vi "InsertNumArrIntoHashTbl.vi"(2 "Hash Table In":refnum<class "HashTable.lvclass">, 3 "Numeric Array In":i32[](array[numeric])) -> (0 "Hash Table Out":refnum<class "HashTable.lvclass">)   [LabVIEW 2021]
uses:
  <vilib>/imath/engines/lvmath2/StdLib/HashTable.llb/HashTable.lvclass
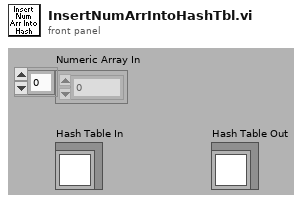
[diagram p1: front panel]
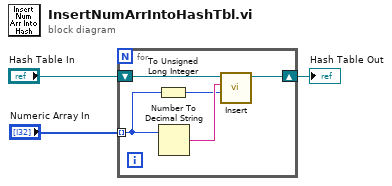
[diagram p0: block diagram]
diagram:
  n1 = for {
    tunnel: "Numeric Array In" -> [w6] mode=indexing
    shift-right: [w5] -> w1
    shift-left: "Hash Table In" -> [w8]
    n2 = To Unsigned Long Integer(number=w6) -> (unsigned 32bit integer=w4:u32)
    n3 = Number To Decimal String(number=w6) -> (decimal integer string=w7:string)  [unwired: 1 out]
    n4 = call <vilib>:"Insert.vi"("Value"=w4, "Key"=w7, "HashTable in"=w8) -> ("HashTable out"=w5:refnum<class "HashTable.lvclass">)  [unwired: 8 out]
  }
  "Hash Table Out" <- w1
